vi "Auto PID Drive.vi"(8 "PID Config":T1 {"Max I Accu"."Low" format="%#.8f"; "Max I Accu"."High" format="%#.8f"; "Gains"."F" format="%#.8f"; "Gains"."D" format="%#.8f"; "Gains"."I" format="%#.8f"; "Gains"."P" format="%#.8f"; "Error Allowed"."Low" format="%#.8f"; "Error Allowed"."High" format="%#.8f"; "I Zone"."Low" format="%#.8f"; "I Zone"."High" format="%#.8f"; "Max Out"."REV" format="%.2f"; "Max Out"."FWD" format="%.2f"}, 9 "Auto Target (ft)":dbl, 10 "Calculated Position (ft)":dbl, 11 "Target Cycle Time(S)":dbl) -> (0 "PID Enabled Out":bool, 1 "Error Out":dbl, 2 "At Target":bool, 3 "Output Out":dbl)   [LabVIEW 2020, in "SwerveDrive_ACT.lvlib"]
uses:
  SwerveDrive_ACT.lvlib
  Shared Code/TypeDefs/Cluster_PID Config.ctl
  Shared Code/TypeDefs/Cluster_PID Gains.ctl
  Shared Code/TypeDefs/Cluster_High-Low.ctl
  Shared Code/TypeDefs/Cluster_FWD  REV Values.ctl
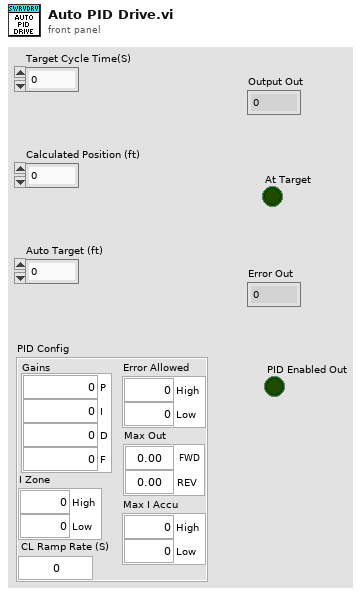
[diagram p1: front panel]
types:
  T1 = typedef "Cluster_PID Config.ctl" = cluster{"Gains":T2, "Error Allowed":T3, "I Zone":T3, "Max Out":T4, "Max I Accu":T3, "CL Ramp Rate (S)":dbl}
  T2 = typedef "Cluster_PID Gains.ctl" = cluster{"P":dbl, "I":dbl, "D":dbl, "F":dbl}
  T3 = typedef "Cluster_High-Low.ctl" = cluster{"High":dbl, "Low":dbl}
  T4 = typedef "Cluster_FWD  REV Values.ctl" = cluster{"FWD":dbl, "REV":dbl}
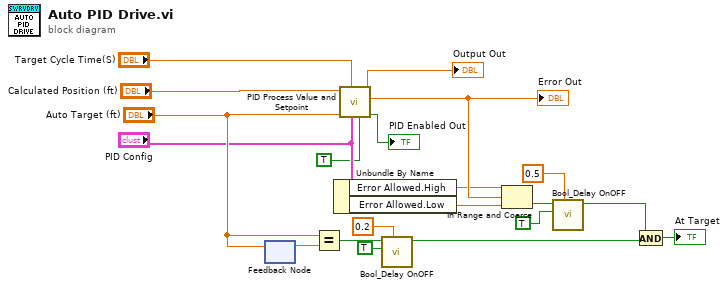
[diagram p0: block diagram]
diagram:
  n1 = feedback #1() -> (w9:dbl)  [unwired: 1 in]
  n2 = feedback-in #1("Auto Target (ft)") -> ()
  n3 = Equal?(x="Auto Target (ft)", y=w9) -> (x = y?=w10:bool)
  n4 = Unbundle By Name("PID Config") -> ("Error Allowed.High"=w6:dbl, "Error Allowed.Low"=w7:dbl)
  n5 = call "PID Process Value and Setpoint.vi"("Allowable Error Disables Accumulator"=TRUE, "PID Config"="PID Config", "Target Cycle Time(S)"="Target Cycle Time(S)", "Setpoint"="Auto Target (ft)", "Process Variable"="Calculated Position (ft)") -> ("PID Enabled Out"=→"PID Enabled Out":bool, "Error Out"=w8:dbl, "Output Out"=→"Output Out":dbl)  [unwired: 3 in, 1 out]
  "Error Out" <- w8
  n6 = call "Bool_Delay OnOFF.vi"("Delay Time(S)"=0.2, "Delay On(t) Off(f)"=TRUE, "Input"=w10) -> ("Output"=w13:bool)  [unwired: 7 in, 1 out]
  n7 = In Range and Coerce(upper limit=w6, x=w8, lower limit=w7) -> (In Range?=w15:bool)  [unwired: 1 out]
  n8 = call "Bool_Delay OnOFF.vi"("Delay Time(S)"=0.5, "Delay On(t) Off(f)"=TRUE, "Input"=w15) -> ("Output"=w18:bool)  [unwired: 7 in, 1 out]
  n9 = And(x=w18, y=w13) -> (x .and. y?=→"At Target":bool)
